vi "TSL235R-Test.vi"() -> ()   [LabVIEW 2013]
panel:
  out "Current Value":dbl
  out "Output Frequency (Hz)":dbl(knob) scale=0.01..1000000.0
  out "Waveform Chart":dbl(graph)
  out "Output Frequency (kHz)":dbl(knob) scale=0.01..1000.0
  in  "Irradiance µW/cm²":dbl(knob) scale=0.001..1000.0
  in  "Stop Button":bool
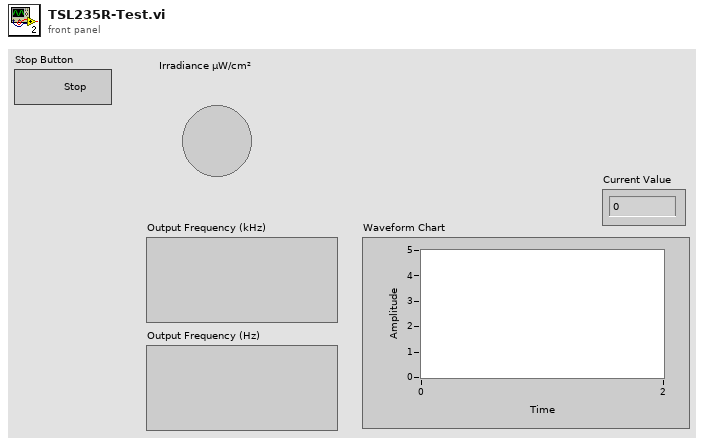
[diagram p1: front panel]
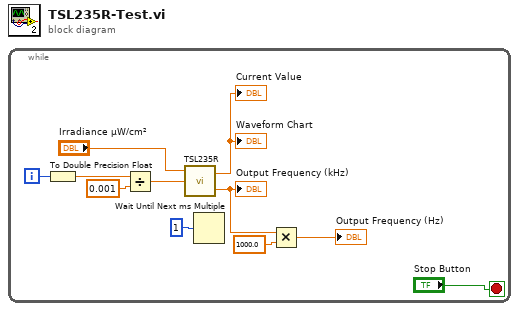
[diagram p0: block diagram]
diagram:
  n1 = while {
    i -> [w6]
    stop <- "Stop Button" stop-if-true
    n2 = To Double Precision Float(number=w6) -> (double precision float=w7:dbl)
    n3 = Divide(x=w7, y=0.001) -> (x/y=w8:dbl)
    n4 = call "TSL235R.vi"("Time s"=w8, "Irradiance µW/cm²"="Irradiance µW/cm²") -> ("Output Frequency (kHz)"=w4:dbl, "Output"=→"Waveform Chart" →"Current Value":dbl)  [unwired: 1 in]
    "Output Frequency (kHz)" <- w4
    n5 = Wait Until Next ms Multiple(millisecond multiple=u32 1) -> ()  [unwired: 1 out]
    n6 = Multiply(x=w4, y=1000.0) -> (x*y=→"Output Frequency (Hz)":dbl)
  }
